vi "BlobDetection.vi"(0 "Color Plane (Color Plane Extraction 1)":i32(ring)=7 items=["Red", "Green", "Blue", "Hue", "Saturation", "Luminance", "Value", "Intensity"], 1 "Method (Threshold 1)":i32(ring)=2 items=["clustering", "entropy", "metric", "moments", "inter-class variance"], 2 "Operation (Basic Morphology 1)":T1(ring)=enum."Dilate", 3 "Min Radius (Circle Detection 1)":sgl=3.0, 4 "Max Radius (Circle Detection 1)":sgl=100.0, 7 "error in":errorcluster) -> (20 "Nb Circles (Circle Detection 1)":i32, 21 "Circles Data (Circle Detection 1)":T3(array[cluster]), 22 "Circles Data (calibrated) (Circle Detection 1)":T3(array[cluster]), 27 "error out":errorcluster)   [LabVIEW 2017]
uses:
  <vilib>/vision/NI_Vision_Development_Module.lvlib
panel:
  out "Image Out":T2(plugin-control)
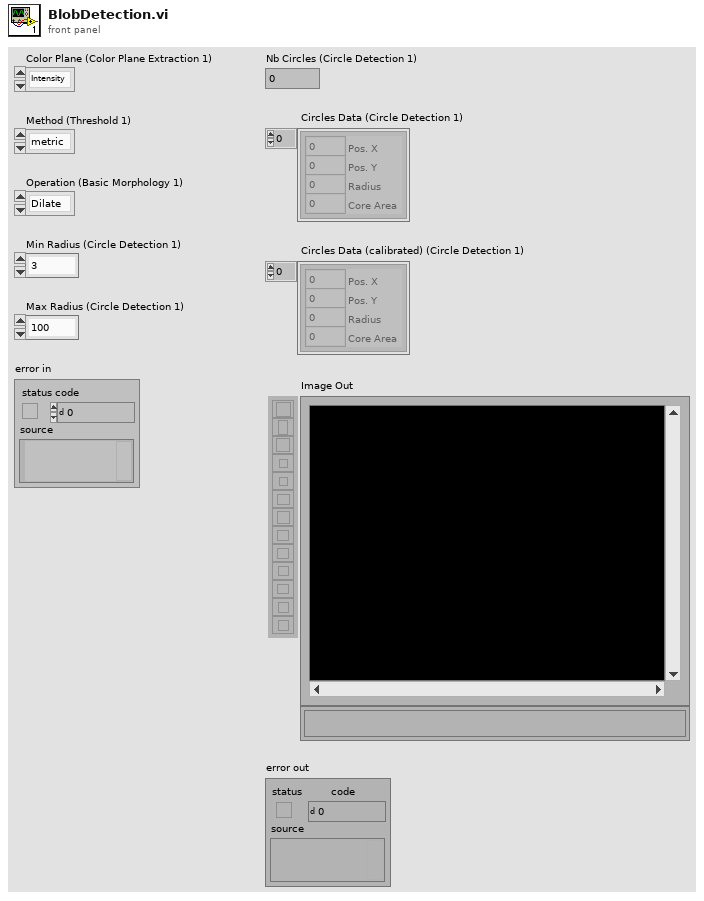
[diagram p1: front panel]
types:
  T1 = enum32{"AutoM", "Close", "Dilate", "Erode", "Gradient", "Gradient out", "Gradient in", "Hit miss", "Open", "PClose", "POpen", "Thick", "Thin"}
  T2 = typedef "IMAQ Image.ctl" = refnum<image>
  T3 = cluster{"Pos. X":i32, "Pos. Y":i32, "Radius":i32, "Core Area":i32}[]
  T4 = typedef "Image Type" = u32
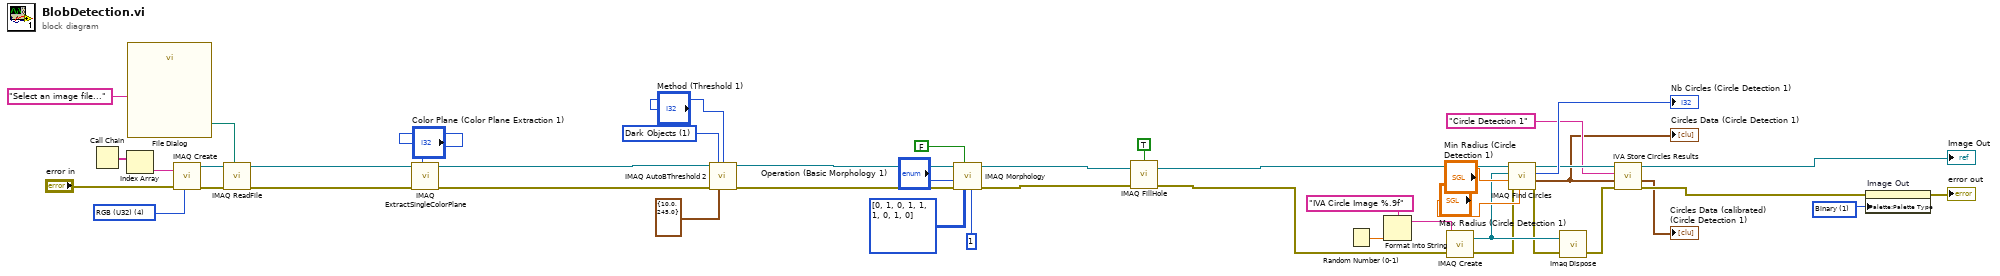
[diagram p0: block diagram]
diagram:
  w1 = u32 1 items=["Grayscale", "Binary", "Gradient", "Rainbow", "Temperature", "User Defined", "Binary 16 Bit", "Gradient 16 Bit", "Rainbow 16 Bit", "Temperature 16 Bit", "User Defined 16 Bit"] ("Palette Type")
  w30 = u32 1 items=["Bright Objects", "Dark Objects"] ("Look For")
  w36 = T4 4 items=["Grayscale (U8)", "Grayscale (I16)", "Grayscale (SGL)", "Complex (CSG)", "RGB (U32)", "HSL (U32)", "RGB (U64)", "Grayscale (U16)"] ("Image Type")
  n1 = Call Chain() -> (call chain=w40:string[])
  n2 = Index Array(array=w40) -> (element=w39:string)  [unwired: 1 in]
  n3 = call "File Dialog"("prompt"="Select an image file...") -> ("selected path"=w37:path)  [unwired: 6 in, 8 out]
  n4 = call "IMAQ Create"("Image Name"=w39, "Image Type"=w36, "error in (no error)"="error in") -> ("New Image"=w43:T2, "error out"=w42:errorcluster)  [unwired: 1 in, 1 out]
  n5 = call "IMAQ ReadFile"("File Path"=w37, "error in (no error)"=w42, "Image"=w43) -> ("error out"=w44:errorcluster, "Image Out"=w34:T2)  [unwired: 2 in, 5 out]
  n6 = call "IMAQ ExtractSingleColorPlane"("Color Plane"="Color Plane (Color Plane Extraction 1)", "error in (no error)"=w44, "Image Src"=w34) -> ("error out"=w33:errorcluster, "Image Dst Out"=w32:T2)  [unwired: 1 in, 6 out]
  n7 = call "IMAQ AutoBThreshold 2"("Image Src"=w32, "Look For (Bright Objects)"=w30, "Method (clustering)"="Method (Threshold 1)", "error in (no error)"=w33, "Threshold Limits"=cluster{"Lower value":sgl, "Upper value":sgl} {"Lower value"=10.0, "Upper value"=245.0}) -> ("Image Dst Out"=w23:T2, "error out"=w31:errorcluster)  [unwired: 3 in, 6 out]
  n8 = call "IMAQ Morphology"("Number of iterations (1)"=1, "Structuring Element"=i32[][] [[0, 1, 0], [1, 1, 1], [0, 1, 0]], "Square/Hexa (Square)"=FALSE, "error in (no error)"=w31, "Operation"="Operation (Basic Morphology 1)", "Image Src"=w23) -> ("error out"=w22:errorcluster, "Image Dst Out"=w20:T2)  [unwired: 1 in, 3 out]
  n9 = call "IMAQ FillHole"("error in (no error)"=w22, "Image Src"=w20, "Connectivity 4/8 (8)"=TRUE) -> ("error out"=w19:errorcluster, "Image Dst Out"=w10:T2)  [unwired: 1 in, 2 out]
  n10 = Random Number (0-1)() -> (number: 0 to 1=w4:dbl)
  n11 = Format Into String(format string="IVA Circle Image %.9f" ("Image Name"), w4) -> (resulting string=w6:string)  [unwired: 2 in, 1 out]
  n12 = call "IMAQ Create"("Image Name"=w6, "error in (no error)"=w19) -> ("New Image"=w15:T2, "error out"=w14:errorcluster)  [unwired: 2 in, 1 out]
  n13 = call "IMAQ Find Circles"("Max Radius"="Max Radius (Circle Detection 1)", "error in (no error)"=w14, "Min Radius"="Min Radius (Circle Detection 1)", "Image Dst"=w15, "Image Src"=w10) -> ("error out"=w13:errorcluster, "Circles Data"=w8:T3, "Nb Circles"=→"Nb Circles (Circle Detection 1)":i32)  [unwired: 4 out]
  "Circles Data (Circle Detection 1)" <- w8
  n14 = call "Imaq Dispose"("Image"=w15, "error in (no error)"=w13) -> ("error out"=w12:errorcluster)  [unwired: 1 in, 3 out]
  n15 = call <vilib>:"IVA Store Circles Results.vi"("error in (no error)"=w12, "Circles Data"=w8, "Step Name"="Circle Detection 1", "Image in"=w10) -> ("error out"=w11:errorcluster, "Circles Data (calibrated)"=→"Circles Data (calibrated) (Circle Detection 1)":T3, "Image dup"=→"Image Out":T2)  [unwired: 5 out]
  n16 = property on="Image Out" class="ImageControl"(error in=w11, "Palette:Palette Type"=w1) -> (error out=→"error out":errorcluster)  [unwired: 1 in, 1 out]
